vi "Align Turret.vi"() -> ()   [LabVIEW 2019]
uses:
  <vilib>/Rock Robotics/WPI/ThirdParty/Phoenix-LabVIEW/Motor Controller/Controls/CTRE_Phoenix_MotorControl_ControlMode.ctl
  Refnums.vi
  <vilib>/Rock Robotics/WPI/ThirdParty/Phoenix-LabVIEW/Motor Controller/Get/CTRE_Phoenix_MotorController_GetQuadratureData.vi
  Global Data.vi
panel:
  out "GTG":bool
  out "EXIT ANGLE":dbl(knob) scale=0.0..90.0
  out "TX ANGLE":dbl(knob) scale=-30.0..30.0
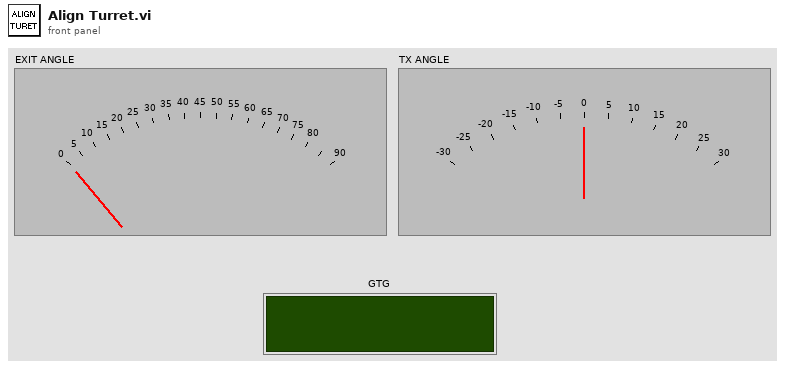
[diagram p1: front panel]
types:
  T1 = typedef "CTRE_Phoenix_MotorControl_ControlMode.ctl" = u16
  T2 = typedef "WPI_RobotDriveDevRef.ctl" = cluster{"DevStatus":errorcluster, "Motors[]":T3[], "Square Inputs":bool, "Max Output":dbl}
  T3 = typedef "WPI_MotorControlDeviceRef.ctl" = cluster{"DeviceStatus":errorcluster, "Type":T4, "PWM":cluster{"PWM Channel":T5, "DeadBand":T6}, "CAN":cluster{"Device Number":u8, "SetOutput VI Ref":variant, "GetOutput VI Ref":variant, "Enable VI Ref":variant, "Disable VI Ref":variant, "Data":variant}, "Invert":bool, "DIO PWM":cluster{"PWM \"Enable\" Channel":T5, "DIOChannel":T7, "PWM Rate":dbl}}
  T4 = typedef "WPI_MotorControlType.ctl" = enum16{"PWM", "CAN", "DIO PWM"}
  T5 = typedef "FPGA_DIOPWMChannel.ctl" = enum8{"PWM 0", "PWM 1", "PWM 2", "PWM 3", "PWM 4", "PWM 5", "PWM 6", "PWM 7", "PWM 8", "PWM 9", "PWM MXP 0", "PWM MXP 1", "PWM MXP 2", "PWM MXP 3", "PWM MXP 4", "PWM MXP 5", "PWM MXP 6", "PWM MXP 7", "PWM MXP 8", "PWM MXP 9", "Invalid"}
  T6 = typedef "WPI_PWMDeadband.ctl" = cluster{"Name":string, "maxPositivePwm":i32, "minPositivePwm":i32, "centerPwm":i32, "maxNegativePwm":i32, "minNegativePwm":i32, "angularRange":u16}
  T7 = typedef "FPGA_DIOChannel.ctl" = enum8{"DIO 0", "DIO 1", "DIO 2", "DIO 3", "DIO 4", "DIO 5", "DIO 6", "DIO 7", "DIO 8", "DIO 9", "DIO MXP 0", "DIO MXP 1", "DIO MXP 2", "DIO MXP 3", "DIO MXP 4", "DIO MXP 5", "DIO MXP 6", "DIO MXP 7", "DIO MXP 8", "DIO MXP 9", "DIO MXP 10", "DIO MXP 11", "DIO MXP 12", "DIO MXP 13", "DIO MXP 14", "DIO MXP 15", "SPI Port CS1", "SPI Port CS2", "SPI Port CS3", "SPI Port MISO", "SPI Port MOSI", "Invalid"}
  T8 = cluster{"ROBOT_DRIVE":T2, "RIGHT_DRIVE":T3, "LEFT_DRIVE":T3, "TURRET":T3, "SHOOTER_MASTER":T3, "HOPPER":T3, "INDEXER":T3, "INTAKE":T3, "CLIMBER_WINCH":T3, "CLIMBER_ARM":T3, "SHOOTER_ANGLE":T3, "SHOOTER_SLAVE":T3}
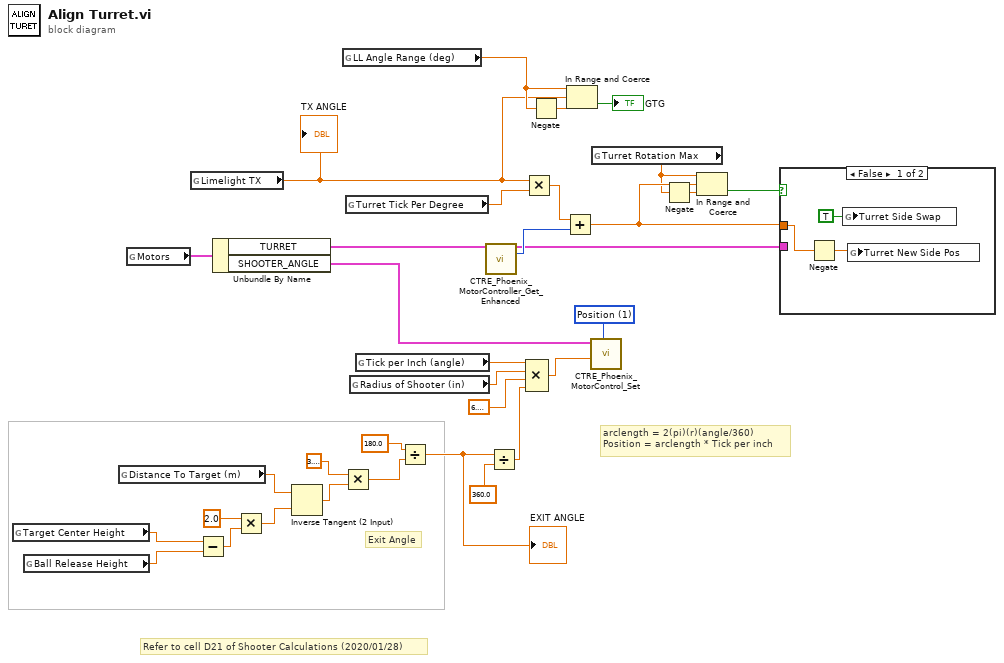
[diagram p0: block diagram]
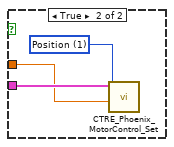
[diagram p2: hidden frame]
diagram:
  w16 = T1 1 items=["PercentOutput"=0, "Position"=1, "Velocity"=2, "Current"=3, "Follower"=5, "MotionProfile"=6, "MotionMagic"=7, "MotionProfileArc"=10, "Disabled"=15] ("Control Mode")
  # "arclength = 2(pi)(r)(angle/360)\nPosition = arclength * Tick per inch"
  # "Exit Angle"
  # "Refer to cell D21 of Shooter Calculations (2020/01/28)"
  n1 = global read "Global Data.vi" "Target Center Height"() -> (w25:dbl)
  n2 = global read "Global Data.vi" "Ball Release Height"() -> (w24:dbl)
  n3 = global read "Global Data.vi" "Distance To Target (m)"() -> (w26:dbl)
  n4 = global read "Refnums.vi" "Motors"() -> (w33:T8)
  n5 = global read "Global Data.vi" "Limelight TX"() -> (w6:dbl)
  "TX ANGLE" <- w6
  n6 = Subtract(x=w25, y=w24) -> (x-y=w23:dbl)
  n7 = Unbundle By Name(w33) -> ("TURRET"=w28:T3, "SHOOTER_ANGLE"=w17:T3)
  n8 = Multiply(x=2.0, y=w23) -> (x*y=w21:dbl)
  n9 = Inverse Tangent (2 Input)(1:w21, 2:w26) -> (0:w20:dbl)
  n10 = global read "Global Data.vi" "LL Angle Range (deg)"() -> (w7:dbl)
  n11 = Multiply(x=3.141592653589793, y=w20) -> (x*y=w18:dbl)
  n12 = global read "Global Data.vi" "Turret Tick Per Degree"() -> (w32:dbl)
  n13 = global read "Global Data.vi" "Radius of Shooter (in)"() -> (w15:dbl)
  n14 = global read "Global Data.vi" "Tick per Inch (angle)"() -> (w11:dbl)
  n15 = Divide(x=180.0, y=w18) -> (x/y=w9:dbl)
  "EXIT ANGLE" <- w9
  n16 = call-poly <vilib>:"CTRE_Phoenix_MotorController_Get_Enhanced.vi"("PhoenixMotorControlDevRef"=w28) -> ("PhoenixMotorControlDevRef"=w29:T3, "Quadrature Position"=w31:i32)  [unwired: 11 in, 2 out]
  n17 = Divide(x=w9, y=360.0) -> (x/y=w13:dbl)
  n18 = Multiply(x=w6, y=w32) -> (x*y=w30:dbl)
  n19 = Compound Arithmetic op=MULTIPLY(w11, w15, 6.283185307179586, w13) -> (w10:dbl)
  n20 = Negate(x=w7) -> (-x=w8:dbl)
  n21 = Add(x=w30, y=w31) -> (x+y=w4:dbl)
  n22 = In Range and Coerce(upper limit=w7, x=w6, lower limit=w8) -> (In Range?=→"GTG":bool)  [unwired: 1 out]
  n23 = call <vilib>:"CTRE_Phoenix_MotorControl_Set.vi"("Output"=w10, "Control Mode"=w16, "PhoenixMotorControlDevRef"=w17) -> ()  [unwired: 7 in, 2 out]
  n24 = global read "Global Data.vi" "Turret Rotation Max"() -> (w2:dbl)
  n25 = Negate(x=w2) -> (-x=w3:dbl)
  n26 = In Range and Coerce(upper limit=w2, x=w4, lower limit=w3) -> (In Range?=w1:bool)  [unwired: 1 out]
  n27 = case shown="False" w1 {
    tunnel: w29 -> [_ w38]
    tunnel: w4 -> [w35 w37]
    frame False {
      n28 = Negate(x=w35) -> (-x=w36:dbl)
      n29 = global write "Global Data.vi" "Turret Side Swap"(TRUE ("Turret Side Swap")) -> ()
      n30 = global write "Global Data.vi" "Turret New Side Pos"(w36) -> ()
    }
    frame True {
      w39 = T1 1 items=["PercentOutput"=0, "Position"=1, "Velocity"=2, "Current"=3, "Follower"=5, "MotionProfile"=6, "MotionMagic"=7, "MotionProfileArc"=10, "Disabled"=15] ("Control Mode")
      n31 = call <vilib>:"CTRE_Phoenix_MotorControl_Set.vi"("Output"=w37, "Control Mode"=w39, "PhoenixMotorControlDevRef"=w38) -> ()  [unwired: 7 in, 2 out]
    }
  }
